vi "pcap-opendev.vi"(0 "Select Device":u32=1 min=1 max=5 step=1) -> (1 "Opened":bool, 2 "Error: \nInvalid Device":bool, 3 "Error:\nOpen Failed":bool)   [LabVIEW 2017]
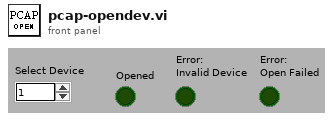
[diagram p1: front panel]
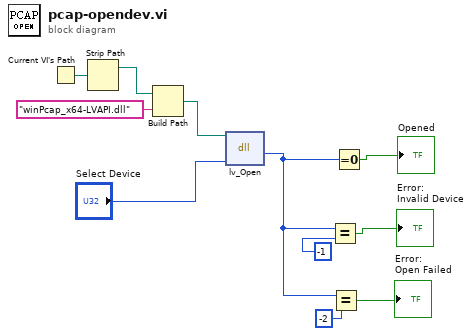
[diagram p0: block diagram]
diagram:
  n1 = Current VI's Path() -> (path=w4:path)
  n2 = Strip Path(path=w4) -> (stripped path=w3:path)  [unwired: 1 out]
  n3 = Build Path(base path=w3, name or relative path="winPcap_x64-LVAPI.dll") -> (appended path=w1:path)
  n4 = dll-call lib="C:/Users/ucbtspu.AD/OneDrive - University College London/Local SCC/SilverLab-Microscope x64/Ethernet/winPcap_x64-LVAPI.dll" fn="lv_Open"(path in=w1, "Select Device") -> ("return type"=w5:i32)  [unwired: 3 in, 2 out]
  n5 = Equal?(x=w5, y=-1) -> (x = y?=→"Error: \nInvalid Device":bool)
  n6 = Equal?(x=w5, y=-2) -> (x = y?=→"Error:\nOpen Failed":bool)
  n7 = Equal To 0?(x=w5) -> (x = 0?=→"Opened":bool)
